vi "Open Session.vi"(8 "error in":errorcluster, 11 "Path":path) -> (0 "error out":errorcluster, 3 "Config Data":refnum<class "Config Data.lvclass">)   [LabVIEW 2014]
uses:
  <vilib>/Utility/config.llb/NI_LVConfig.lvlib
  Config Data.lvclass
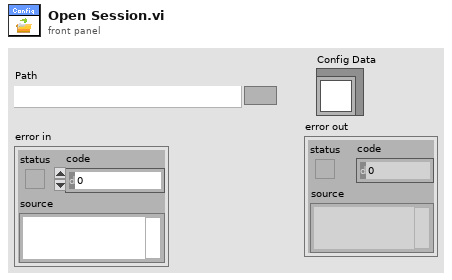
[diagram p1: front panel]
types:
  T1 = typedef "NI_LVConfig.lvlib/Config Data RefNum.ctl" = refnum<k1>
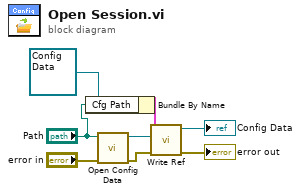
[diagram p0: block diagram]
diagram:
  n1 = Bundle By Name(cluster=refnum<class "Config Data.lvclass"> refnum ("Config Data"), "Cfg Path"="Path") -> (w2:cluster{})
  n2 = call <vilib>:"Open Config Data.vi"("error in (no error)"="error in", "configuration file path"="Path") -> ("error out"=w6:errorcluster, "refnum"=w8:T1)  [unwired: 7 in, 1 out]
  n3 = call "Write Ref.vi"("error in (no error)"=w6, "config data"=w8, "Config Data in"=w2) -> ("error out"=→"error out":errorcluster, "Config Data out"=→"Config Data":refnum<class "Config Data.lvclass">)  [unwired: 7 in]
